vi "Connect TCP.vi"(6 "timeout (100ms)":i32=100, 8 "error in (no error)":errorcluster, 10 "remote port (80)":u16=80, 11 "address (localhost)":string="localhost") -> (0 "error out":errorcluster, 3 "TCPConnection":refnum<class "TCPConnection.lvclass">)   [LabVIEW 2013, in "MQTT_TCP.lvlib" / "TCPConnection.lvclass"]
uses:
  TCPConnection.lvclass
  TCPConnection.lvclass/TCPConnection.ctl
  <vilib>/LabVIEW Open Source Project/MQTT Connection/MQTT_Connection/Connection/Connection.lvclass/Connection.ctl
  <vilib>/LabVIEW Open Source Project/MQTT Connection/MQTT_Connection/Connection/Connection.lvclass
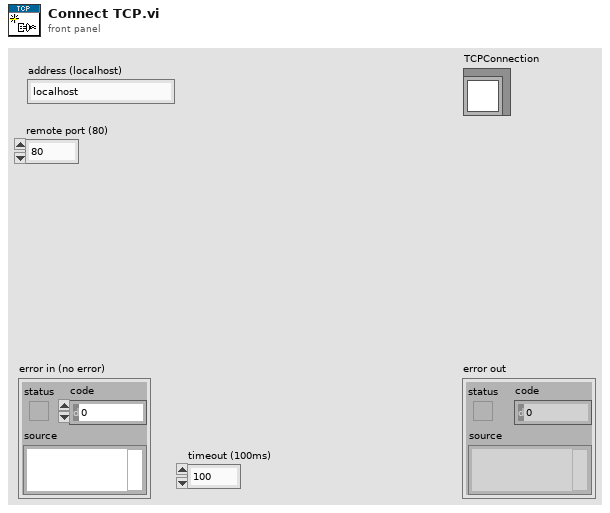
[diagram p1: front panel]
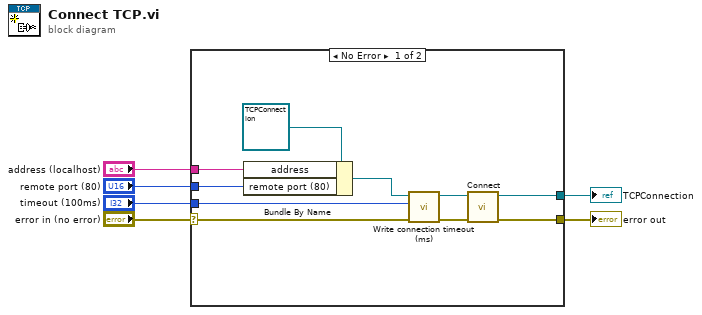
[diagram p0: block diagram]
diagram:
  n1 = case shown="No Error" "error in (no error)" {
    selector: "error in (no error)" -> [w9 w17]
    tunnel: [w12 w17] -> w5
    tunnel: [w13 _] -> w1
    tunnel: "address (localhost)" -> [w15 _]
    tunnel: "remote port (80)" -> [w14 _]
    tunnel: "timeout (100ms)" -> [w7 _]
    frame No Error {
      n2 = Bundle By Name(cluster=refnum<class "TCPConnection.lvclass"> refnum ("TCPConnection in"), "address"=w15, "remote port (80)"=w14) -> (w11:refnum<class "TCPConnection.lvclass">)
      n3 = call <vilib>:"Write connection timeout (ms).vi"("error in (no error)"=w9, "connection timeout (ms)"=w7, "Connection in"=w11) -> ("error out"=w8:errorcluster, "Connection out"=w10:refnum<class "TCPConnection.lvclass">)  [unwired: 7 in]
      n4 = call <vilib>:"Connect.vi"("error in (no error)"=w8, "Connection in"=w10) -> ("error out"=w12:errorcluster, "Connection out"=w13:refnum<class "TCPConnection.lvclass">)  [unwired: 8 in]
    }
    frame Error {
    }
  }
  "error out" <- w5
  "TCPConnection" <- w1
